vi "practica1_2.4.vi"() -> ()   [LabVIEW 2016]
panel:
  out "ans":string
  in  "division":bool
  in  "multiplicacion":bool
  in  "resta":bool
  in  "suma":bool
  in  "segundo numero":dbl
  in  "primer numero":dbl
  # "esta calculadora funciona poniendo los numeros y luego seleccionas\nla operacion si presionas mas de una aparceceran todos los mensajes \nde los resultados en ans"
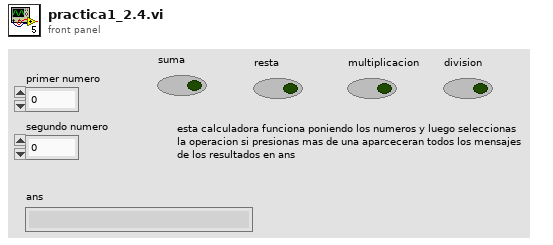
[diagram p1: front panel]
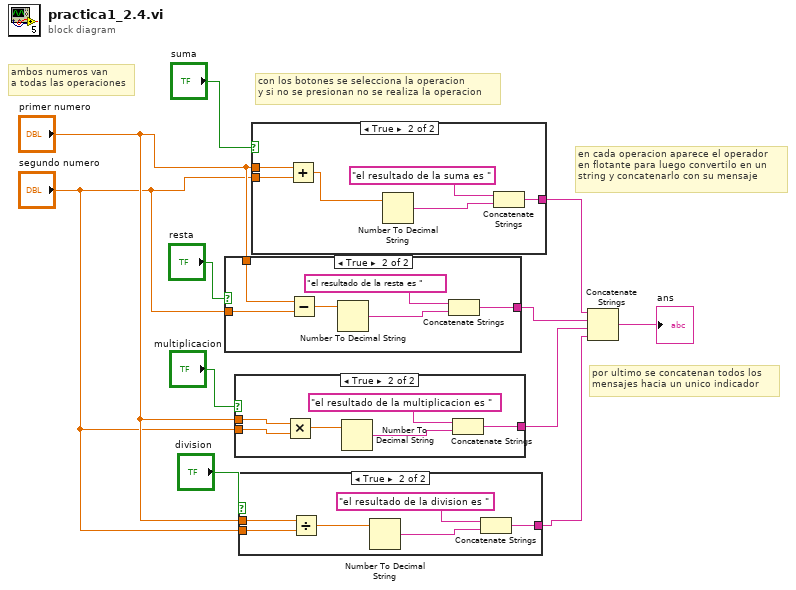
[diagram p0: block diagram]
diagram:
  # "por ultimo se concatenan todos los\nmensajes hacia un unico indicador"
  # "en cada operacion aparece el operador \nen flotante para luego convertilo en un \nstring y concatenarlo con su mensaje"
  # "ambos numeros van \na todas las operaciones"
  # "con los botones se selecciona la operacion\ny si no se presionan no se realiza la operacion"
  n1 = case shown="True" "resta" {
    tunnel: "primer numero" -> [_ w17]
    tunnel: "segundo numero" -> [_ w16]
    tunnel: [_ w12] -> w4
    frame False {
    }
    frame True {
      n2 = Subtract(x=w17, y=w16) -> (x-y=w13:dbl)
      n3 = Number To Decimal String(number=w13) -> (decimal integer string=w14:string)  [unwired: 1 in]
      n4 = Concatenate Strings("el resultado de la resta es ", w14) -> (w12:string)
    }
  }
  n5 = case shown="True" "multiplicacion" {
    tunnel: "primer numero" -> [_ w23]
    tunnel: "segundo numero" -> [_ w22]
    tunnel: [_ w18] -> w3
    frame False {
    }
    frame True {
      n6 = Multiply(x=w23, y=w22) -> (x*y=w19:dbl)
      n7 = Number To Decimal String(number=w19) -> (decimal integer string=w20:string)  [unwired: 1 in]
      n8 = Concatenate Strings("el resultado de la multiplicacion es ", w20) -> (w18:string)
    }
  }
  n9 = case shown="True" "division" {
    tunnel: "primer numero" -> [_ w29]
    tunnel: "segundo numero" -> [_ w28]
    tunnel: [_ w24] -> w2
    frame False {
    }
    frame True {
      n10 = Divide(x=w29, y=w28) -> (x/y=w25:dbl)
      n11 = Number To Decimal String(number=w25) -> (decimal integer string=w26:string)  [unwired: 1 in]
      n12 = Concatenate Strings("el resultado de la division es ", w26) -> (w24:string)
    }
  }
  n13 = case shown="True" "suma" {
    tunnel: "primer numero" -> [_ w35]
    tunnel: "segundo numero" -> [_ w34]
    tunnel: [_ w30] -> w5
    frame False {
    }
    frame True {
      n14 = Add(x=w35, y=w34) -> (x+y=w31:dbl)
      n15 = Number To Decimal String(number=w31) -> (decimal integer string=w32:string)  [unwired: 1 in]
      n16 = Concatenate Strings("el resultado de la suma es ", w32) -> (w30:string)
    }
  }
  n17 = Concatenate Strings(w5, w4, w3, w2) -> (→"ans":string)
